vi "Expected Vertex Order.vi"(11 "Draw Mode":T1(ring)) -> (3 "Picture":picture)   [LabVIEW 2016]
doc: "Create a picture to illustrate how the mesh would use vertices to generate the 3D picture."
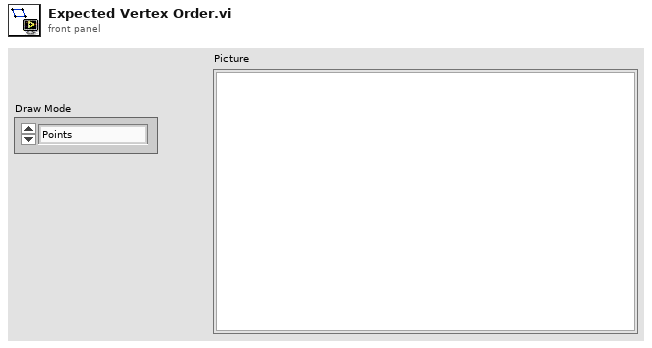
[diagram p1: front panel]
types:
  T1 = enum16{"Points", "Lines", "Line Strip", "Line Loop", "Triangles", "Triangle Strip", "Triangle Fan", "Quads", "Quad Strip", "Polygon"}
  T2 = enum16{"User-specified Font", "Application Font", "System Font", "Dialog Font"}
  T3 = cluster{"Font Name:":string, "Size":i16, "Strikeout?":bool, "Italic?":bool, "Underline?":bool, "Outline?":bool, "Shadow?":bool, "Bold?":bool}
  T4 = cluster{"Width":u16, "Style":enum32{"Solid", "Dash", "Dot", "DashDot", "DashDotDot"}}
  T5 = cluster{"horizontal":enum16{"left", "center", "right"}, "vertical":enum16{"top", "center", "bottom"}}
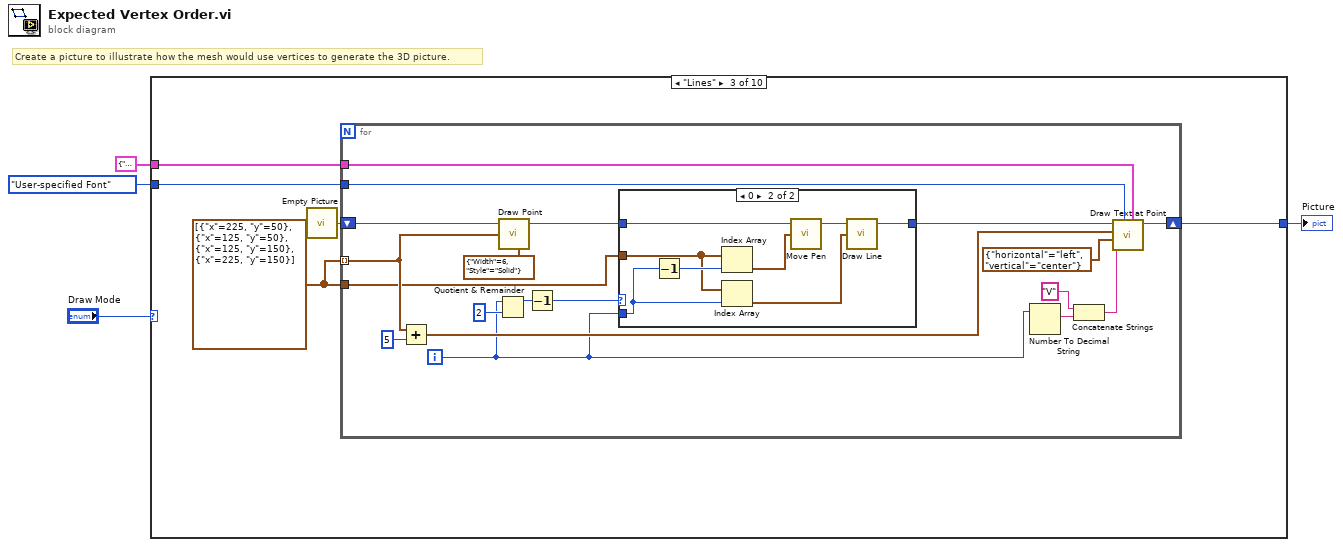
[diagram p0: block diagram]
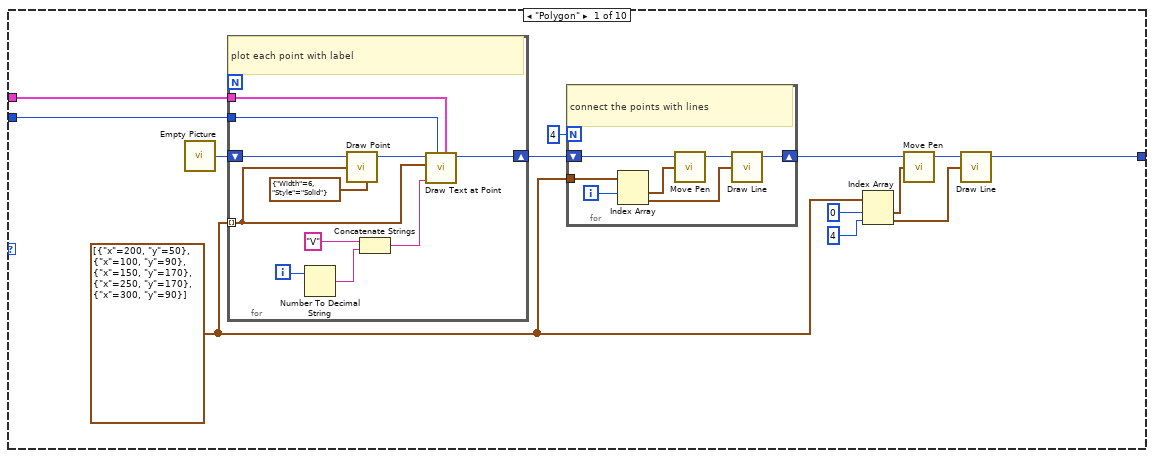
[diagram p2: hidden frame]
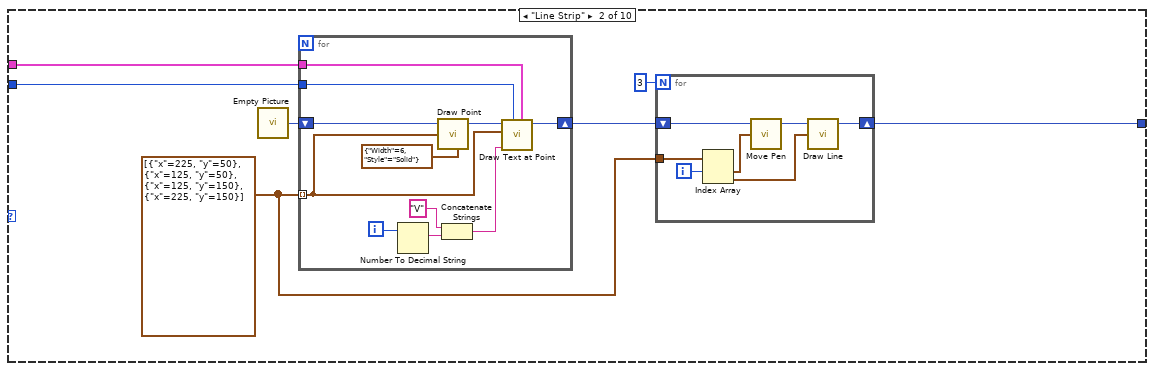
[diagram p3: hidden frame]
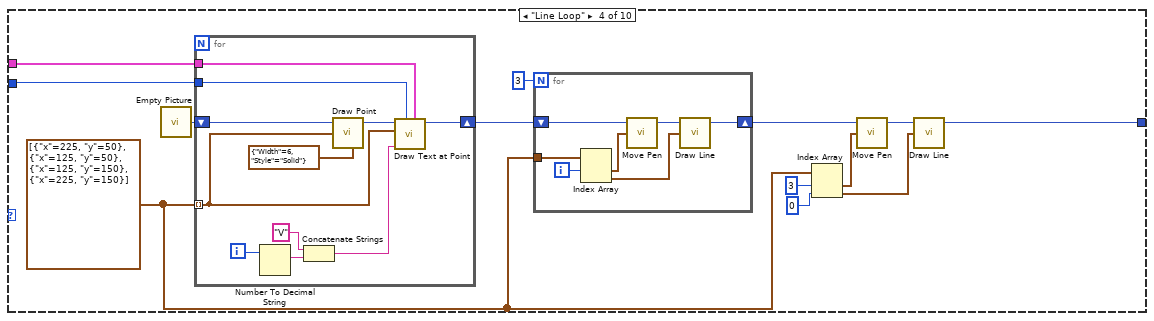
[diagram p5: hidden frame]
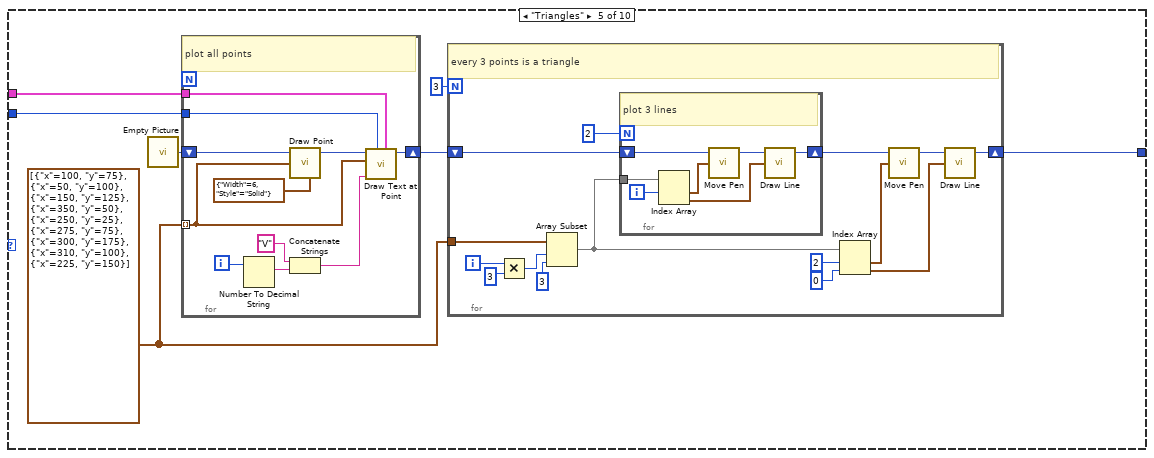
[diagram p6: hidden frame]
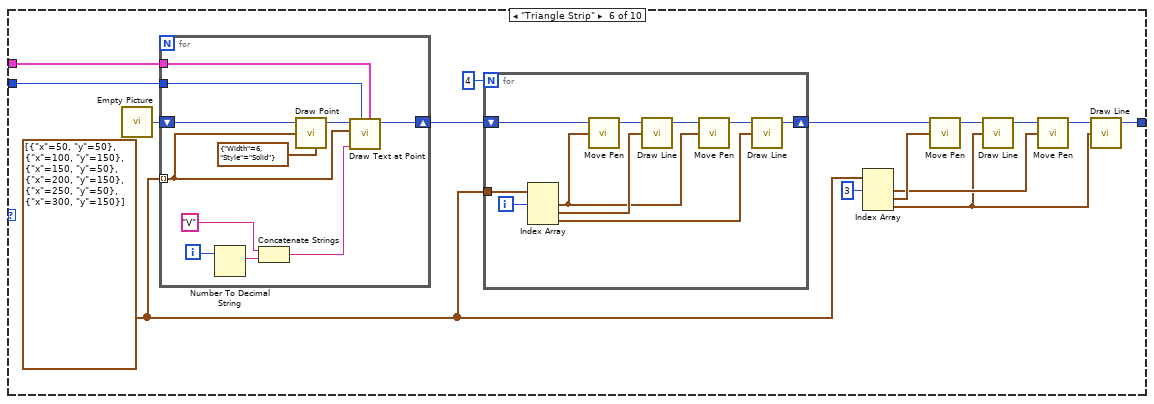
[diagram p7: hidden frame]
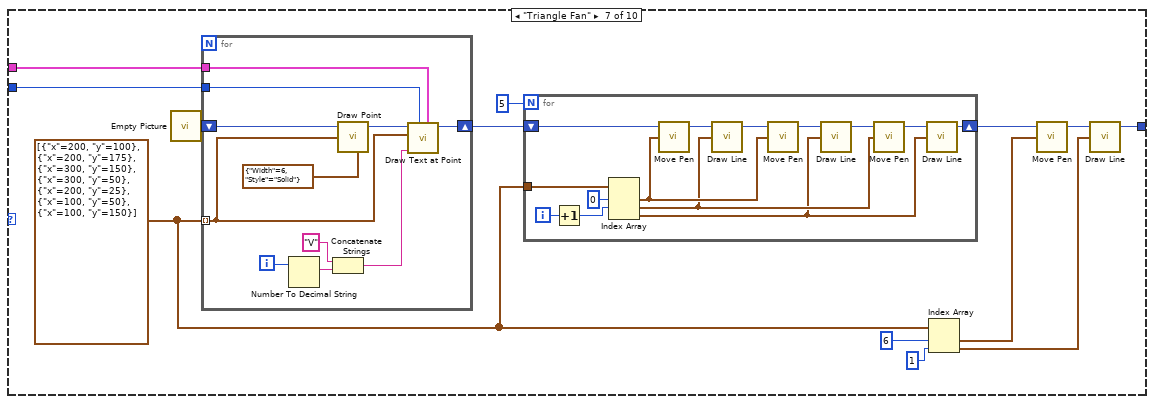
[diagram p8: hidden frame]
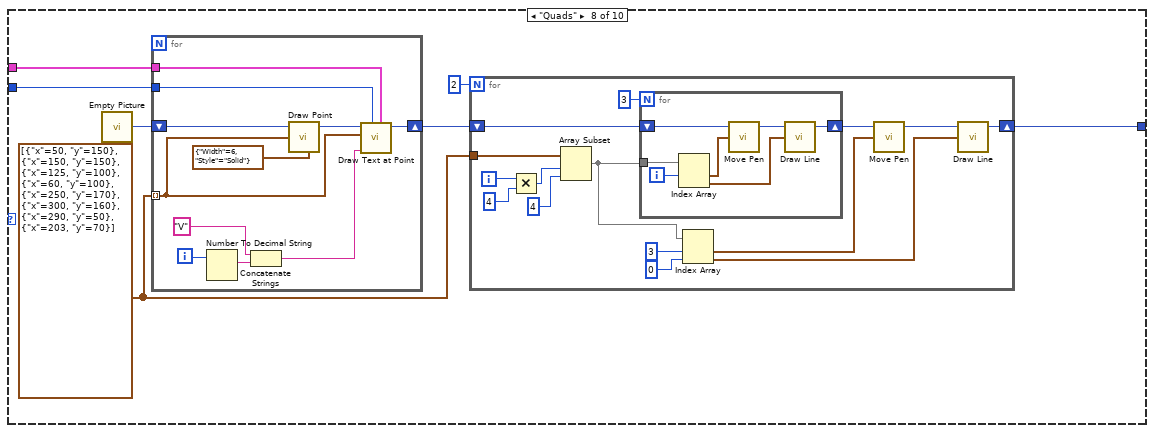
[diagram p9: hidden frame]
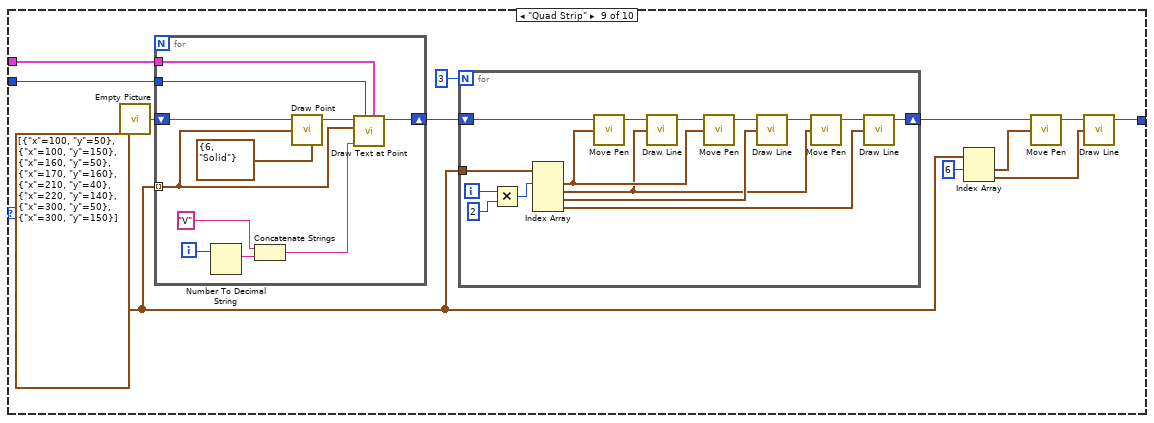
[diagram p10: hidden frame]
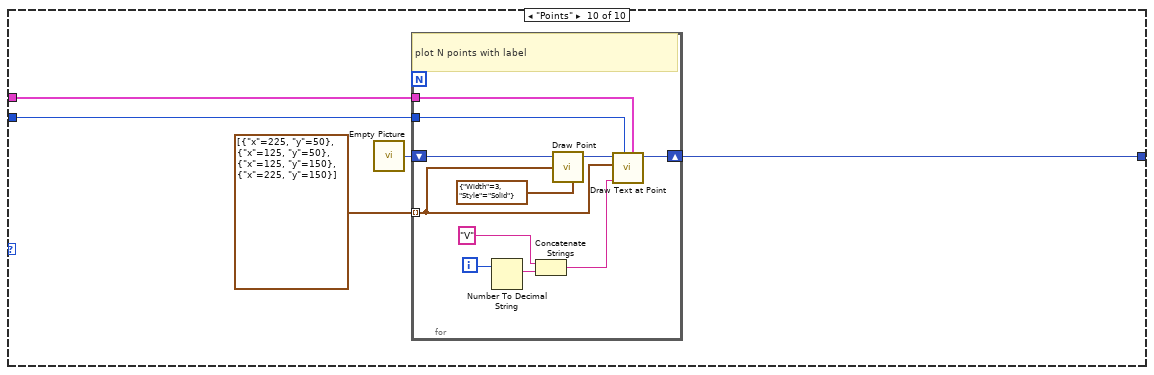
[diagram p11: hidden frame]
diagram:
  # "Create a picture to illustrate how the mesh would use vertices to generate the 3D picture."
  n1 = case shown="\"Lines\"" "Draw Mode" {
    tunnel: [w7 w38 w64 w101 w127 w170 w208 w241 w282 w320] -> w3
    tunnel: T3 {"Font Name:"="Courier", "Size"=15, "Strikeout?"=FALSE, "Italic?"=FALSE, "Underline?"=FALSE, "Outline?"=FALSE, "Shadow?"=FALSE, "Bold?"=TRUE} ("[user-specified font]") -> [w6 w36 w62 w94 w126 w165 w202 w240 w281 w317]
    tunnel: T2."User-specified Font" ("desired font(Application)") -> [w5 w37 w61 w95 w125 w166 w203 w239 w280 w318]
    frame "Polygon" {
      w10 = cluster{"x":i16, "y":i16}[] [{"x"=200, "y"=50}, {"x"=100, "y"=90}, {"x"=150, "y"=170}, {"x"=250, "y"=170}, {"x"=300, "y"=90}]
      n2 = call "Empty Picture"() -> ("empty picture"=w17:picture)
      n3 = for {
        tunnel: w10 -> [w35] mode=indexing
        shift-right: [w27] -> w15
        shift-left: w17 -> [w29]
        tunnel: w6 -> [w26]
        tunnel: w5 -> [w25]
        i -> [w33]
        # "plot each point with label"
        n4 = Number To Decimal String(number=w33) -> (decimal integer string=w32:string)  [unwired: 1 in]
        n5 = call <vilib>:"Draw Point.vi"("picture"=w29, "point(x,y)"=w35, "pen"=T4 {"Width"=6, "Style"=enum."Solid"}) -> ("new picture"=w28:picture)  [unwired: 6 in]
        n6 = Concatenate Strings("V", w32) -> (w30:string)
        n7 = call <vilib>:"Draw Text at Point.vi"("[user-specified font]"=w26, "desired font(Application)"=w25, "text"=w30, "origin"=w35, "picture"=w28) -> ("new picture"=w27:picture)  [unwired: 5 in, 1 out]
      }
      n8 = for {
        N: 4 -> [_]
        shift-right: [w20] -> w11
        shift-left: w15 -> [w21]
        tunnel: w10 -> [w19]
        i -> [w18]
        # "connect the points with lines"
        n9 = Index Array(array=w19, index #1=w18) -> (element #1=w24:cluster{"x":i16, "y":i16}, element #2=w23:cluster{"x":i16, "y":i16})  [unwired: 1 in]
        n10 = call <vilib>:"Move Pen.vi"("new position"=w24, "picture"=w21) -> ("new picture"=w22:picture)  [unwired: 3 in]
        n11 = call <vilib>:"Draw Line.vi"("picture"=w22, "end point"=w23) -> ("new picture"=w20:picture)  [unwired: 7 in]
      }
      n12 = Index Array(array=w10, index #1=0 ("index"), index #2=4 ("index")) -> (element #1=w12:cluster{"x":i16, "y":i16}, element #2=w13:cluster{"x":i16, "y":i16})
      n13 = call <vilib>:"Move Pen.vi"("new position"=w12, "picture"=w11) -> ("new picture"=w14:picture)  [unwired: 3 in]
      n14 = call <vilib>:"Draw Line.vi"("picture"=w14, "end point"=w13) -> ("new picture"=w7:picture)  [unwired: 7 in]
    }
    frame "Line Strip" {
      w39 = cluster{"x":i16, "y":i16}[] [{"x"=225, "y"=50}, {"x"=125, "y"=50}, {"x"=125, "y"=150}, {"x"=225, "y"=150}]
      n15 = call "Empty Picture"() -> ("empty picture"=w42:picture)
      n16 = for {
        tunnel: w39 -> [w60] mode=indexing
        shift-right: [w52] -> w41
        shift-left: w42 -> [w54]
        tunnel: w37 -> [w51]
        tunnel: w36 -> [w50]
        i -> [w58]
        n17 = Number To Decimal String(number=w58) -> (decimal integer string=w57:string)  [unwired: 1 in]
        n18 = call <vilib>:"Draw Point.vi"("picture"=w54, "point(x,y)"=w60, "pen"=T4 {"Width"=6, "Style"=enum."Solid"}) -> ("new picture"=w53:picture)  [unwired: 6 in]
        n19 = Concatenate Strings("V", w57) -> (w55:string)
        n20 = call <vilib>:"Draw Text at Point.vi"("[user-specified font]"=w50, "desired font(Application)"=w51, "text"=w55, "origin"=w60, "picture"=w53) -> ("new picture"=w52:picture)  [unwired: 5 in, 1 out]
      }
      n21 = for {
        N: 3 -> [_]
        shift-right: [w43] -> w38
        shift-left: w41 -> [w44]
        tunnel: w39 -> [w48]
        i -> [w49]
        n22 = Index Array(array=w48, index #1=w49) -> (element #1=w47:cluster{"x":i16, "y":i16}, element #2=w46:cluster{"x":i16, "y":i16})  [unwired: 1 in]
        n23 = call <vilib>:"Move Pen.vi"("new position"=w47, "picture"=w44) -> ("new picture"=w45:picture)  [unwired: 3 in]
        n24 = call <vilib>:"Draw Line.vi"("picture"=w45, "end point"=w46) -> ("new picture"=w43:picture)  [unwired: 7 in]
      }
    }
    frame "Lines" {
      w63 = cluster{"x":i16, "y":i16}[] [{"x"=225, "y"=50}, {"x"=125, "y"=50}, {"x"=125, "y"=150}, {"x"=225, "y"=150}]
      n25 = call "Empty Picture"() -> ("empty picture"=w65:picture)
      n26 = for {
        tunnel: w63 -> [w84] mode=indexing
        shift-right: [w78] -> w64
        shift-left: w65 -> [w79]
        tunnel: w63 -> [w72]
        tunnel: w62 -> [w68]
        tunnel: w61 -> [w67]
        i -> [w71]
        n27 = Add(x=w84, y=5) -> (x+y=w75:cluster{"x":i32, "y":i32})
        n28 = Quotient & Remainder(x=w71, y=2) -> (x-y*floor(x/y)=w73:i32)  [unwired: 1 out]
        n29 = call <vilib>:"Draw Point.vi"("picture"=w79, "point(x,y)"=w84, "pen"=T4 {"Width"=6, "Style"=enum."Solid"}) -> ("new picture"=w70:picture)  [unwired: 6 in]
        n30 = Decrement(x=w73) -> (x-1=w66:i32)
        n31 = case shown="0" w66 {
          tunnel: w72 -> [_ w90]
          tunnel: w71 -> [_ w89]
          tunnel: w70 -> [w85 w91]
          tunnel: [w85 w86] -> w69
          frame Default {
          }
          frame 0 {
            n32 = Decrement(x=w89) -> (x-1=w93:i32)
            n33 = Index Array(array=w90, index=w93) -> (element=w92:cluster{"x":i16, "y":i16})
            n34 = Index Array(array=w90, index=w89) -> (element=w88:cluster{"x":i16, "y":i16})
            n35 = call <vilib>:"Move Pen.vi"("new position"=w92, "picture"=w91) -> ("new picture"=w87:picture)  [unwired: 3 in]
            n36 = call <vilib>:"Draw Line.vi"("picture"=w87, "end point"=w88) -> ("new picture"=w86:picture)  [unwired: 7 in]
          }
        }
        n37 = Number To Decimal String(number=w71) -> (decimal integer string=w82:string)  [unwired: 1 in]
        n38 = Concatenate Strings("V", w82) -> (w80:string)
        n39 = call <vilib>:"Draw Text at Point.vi"("[user-specified font]"=w68, "desired font(Application)"=w67, "text"=w80, "alignment(left, top)"=T5 {"horizontal"=enum."left", "vertical"=enum."center"}, "origin"=w75, "picture"=w69) -> ("new picture"=w78:picture)  [unwired: 4 in, 1 out]
      }
    }
    frame "Line Loop" {
      w98 = cluster{"x":i16, "y":i16}[] [{"x"=225, "y"=50}, {"x"=125, "y"=50}, {"x"=125, "y"=150}, {"x"=225, "y"=150}]
      n40 = call "Empty Picture"() -> ("empty picture"=w106:picture)
      n41 = for {
        tunnel: w98 -> [w124] mode=indexing
        shift-right: [w116] -> w104
        shift-left: w106 -> [w118]
        tunnel: w95 -> [w115]
        tunnel: w94 -> [w114]
        i -> [w122]
        n42 = Number To Decimal String(number=w122) -> (decimal integer string=w121:string)  [unwired: 1 in]
        n43 = Concatenate Strings("V", w121) -> (w119:string)
        n44 = call <vilib>:"Draw Point.vi"("picture"=w118, "point(x,y)"=w124, "pen"=T4 {"Width"=6, "Style"=enum."Solid"}) -> ("new picture"=w117:picture)  [unwired: 6 in]
        n45 = call <vilib>:"Draw Text at Point.vi"("[user-specified font]"=w114, "desired font(Application)"=w115, "text"=w119, "origin"=w124, "picture"=w117) -> ("new picture"=w116:picture)  [unwired: 5 in, 1 out]
      }
      n46 = for {
        N: 3 -> [_]
        shift-right: [w107] -> w102
        shift-left: w104 -> [w108]
        tunnel: w98 -> [w112]
        i -> [w113]
        n47 = Index Array(array=w112, index #1=w113) -> (element #1=w111:cluster{"x":i16, "y":i16}, element #2=w110:cluster{"x":i16, "y":i16})  [unwired: 1 in]
        n48 = call <vilib>:"Move Pen.vi"("new position"=w111, "picture"=w108) -> ("new picture"=w109:picture)  [unwired: 3 in]
        n49 = call <vilib>:"Draw Line.vi"("picture"=w109, "end point"=w110) -> ("new picture"=w107:picture)  [unwired: 7 in]
      }
      n50 = Index Array(array=w98, index #1=3 ("index"), index #2=0 ("index")) -> (element #1=w97:cluster{"x":i16, "y":i16}, element #2=w96:cluster{"x":i16, "y":i16})
      n51 = call <vilib>:"Move Pen.vi"("new position"=w97, "picture"=w102) -> ("new picture"=w103:picture)  [unwired: 3 in]
      n52 = call <vilib>:"Draw Line.vi"("picture"=w103, "end point"=w96) -> ("new picture"=w101:picture)  [unwired: 7 in]
    }
    frame "Triangles" {
      w129 = cluster{"x":i16, "y":i16}[] [{"x"=100, "y"=75}, {"x"=50, "y"=100}, {"x"=150, "y"=125}, {"x"=350, "y"=50}, {"x"=250, "y"=25}, {"x"=275, "y"=75}, {"x"=300, "y"=175}, {"x"=310, "y"=100}, {"x"=225, "y"=150}]
      n53 = call "Empty Picture"() -> ("empty picture"=w131:picture)
      n54 = for {
        tunnel: w129 -> [w164] mode=indexing
        shift-right: [w156] -> w128
        shift-left: w131 -> [w158]
        tunnel: w126 -> [w155]
        tunnel: w125 -> [w154]
        i -> [w162]
        # "plot all points"
        n55 = Number To Decimal String(number=w162) -> (decimal integer string=w161:string)  [unwired: 1 in]
        n56 = call <vilib>:"Draw Point.vi"("picture"=w158, "point(x,y)"=w164, "pen"=T4 {"Width"=6, "Style"=enum."Solid"}) -> ("new picture"=w157:picture)  [unwired: 6 in]
        n57 = Concatenate Strings("V", w161) -> (w159:string)
        n58 = call <vilib>:"Draw Text at Point.vi"("[user-specified font]"=w155, "desired font(Application)"=w154, "text"=w159, "origin"=w164, "picture"=w157) -> ("new picture"=w156:picture)  [unwired: 5 in, 1 out]
      }
      n59 = for {
        N: 3 -> [_]
        tunnel: w129 -> [w143]
        shift-right: [w133] -> w127
        shift-left: w128 -> [w140]
        i -> [w146]
        # "every 3 points is a triangle"
        n60 = Multiply(x=w146, y=3) -> (x*y=w144:i32)
        n61 = Array Subset(array=w143, index=w144, length=3) -> (w139:cluster{"x":i16, "y":i16}[])
        n62 = for {
          N: 2 -> [_]
          tunnel: w139 -> [w153]
          shift-right: [w147] -> w136
          shift-left: w140 -> [w148]
          i -> [w152]
          # "plot 3 lines"
          n63 = Index Array(array=w153, index #1=w152) -> (element #1=w151:cluster{"x":i16, "y":i16}, element #2=w149:cluster{"x":i16, "y":i16})  [unwired: 1 in]
          n64 = call <vilib>:"Move Pen.vi"("new position"=w151, "picture"=w148) -> ("new picture"=w150:picture)  [unwired: 3 in]
          n65 = call <vilib>:"Draw Line.vi"("picture"=w150, "end point"=w149) -> ("new picture"=w147:picture)  [unwired: 7 in]
        }
        n66 = Index Array(array=w139, index #1=2 ("index"), index #2=0 ("index")) -> (element #1=w135:cluster{"x":i16, "y":i16}, element #2=w134:cluster{"x":i16, "y":i16})
        n67 = call <vilib>:"Move Pen.vi"("new position"=w135, "picture"=w136) -> ("new picture"=w137:picture)  [unwired: 3 in]
        n68 = call <vilib>:"Draw Line.vi"("picture"=w137, "end point"=w134) -> ("new picture"=w133:picture)  [unwired: 7 in]
      }
    }
    frame "Triangle Strip" {
      w174 = cluster{"x":i16, "y":i16}[] [{"x"=50, "y"=50}, {"x"=100, "y"=150}, {"x"=150, "y"=50}, {"x"=200, "y"=150}, {"x"=250, "y"=50}, {"x"=300, "y"=150}]
      n69 = call "Empty Picture"() -> ("empty picture"=w179:picture)
      n70 = for {
        tunnel: w174 -> [w200] mode=indexing
        shift-right: [w192] -> w177
        shift-left: w179 -> [w194]
        tunnel: w166 -> [w191]
        tunnel: w165 -> [w190]
        i -> [w198]
        n71 = Number To Decimal String(number=w198) -> (decimal integer string=w197:string)  [unwired: 1 in]
        n72 = Concatenate Strings("V", w197) -> (w195:string)
        n73 = call <vilib>:"Draw Point.vi"("picture"=w194, "point(x,y)"=w200, "pen"=T4 {"Width"=6, "Style"=enum."Solid"}) -> ("new picture"=w193:picture)  [unwired: 6 in]
        n74 = call <vilib>:"Draw Text at Point.vi"("[user-specified font]"=w190, "desired font(Application)"=w191, "text"=w195, "origin"=w200, "picture"=w193) -> ("new picture"=w192:picture)  [unwired: 5 in, 1 out]
      }
      n75 = for {
        N: 4 -> [_]
        shift-right: [w181] -> w175
        shift-left: w177 -> [w187]
        tunnel: w174 -> [w189]
        i -> [w188]
        n76 = Index Array(array=w189, index #1=w188) -> (element #1=w183:cluster{"x":i16, "y":i16}, element #2=w185:cluster{"x":i16, "y":i16}, element #3=w180:cluster{"x":i16, "y":i16})  [unwired: 2 in]
        n77 = call <vilib>:"Move Pen.vi"("new position"=w183, "picture"=w187) -> ("new picture"=w186:picture)  [unwired: 3 in]
        n78 = call <vilib>:"Draw Line.vi"("picture"=w186, "end point"=w185) -> ("new picture"=w184:picture)  [unwired: 7 in]
        n79 = call <vilib>:"Move Pen.vi"("new position"=w183, "picture"=w184) -> ("new picture"=w182:picture)  [unwired: 3 in]
        n80 = call <vilib>:"Draw Line.vi"("picture"=w182, "end point"=w180) -> ("new picture"=w181:picture)  [unwired: 7 in]
      }
      n81 = Index Array(array=w174, index #1=3 ("index")) -> (element #1=w168:cluster{"x":i16, "y":i16}, element #2=w172:cluster{"x":i16, "y":i16}, element #3=w167:cluster{"x":i16, "y":i16})  [unwired: 2 in]
      n82 = call <vilib>:"Move Pen.vi"("new position"=w172, "picture"=w175) -> ("new picture"=w176:picture)  [unwired: 3 in]
      n83 = call <vilib>:"Draw Line.vi"("picture"=w176, "end point"=w167) -> ("new picture"=w169:picture)  [unwired: 7 in]
      n84 = call <vilib>:"Move Pen.vi"("new position"=w168, "picture"=w169) -> ("new picture"=w171:picture)  [unwired: 3 in]
      n85 = call <vilib>:"Draw Line.vi"("picture"=w171, "end point"=w167) -> ("new picture"=w170:picture)  [unwired: 7 in]
    }
    frame "Triangle Fan" {
      w201 = cluster{"x":i16, "y":i16}[] [{"x"=200, "y"=100}, {"x"=200, "y"=175}, {"x"=300, "y"=150}, {"x"=300, "y"=50}, {"x"=200, "y"=25}, {"x"=100, "y"=50}, {"x"=100, "y"=150}]
      n86 = call "Empty Picture"() -> ("empty picture"=w213:picture)
      n87 = for {
        tunnel: w201 -> [w238] mode=indexing
        shift-right: [w230] -> w212
        shift-left: w213 -> [w232]
        tunnel: w203 -> [w229]
        tunnel: w202 -> [w228]
        i -> [w236]
        n88 = Number To Decimal String(number=w236) -> (decimal integer string=w235:string)  [unwired: 1 in]
        n89 = Concatenate Strings("V", w235) -> (w233:string)
        n90 = call <vilib>:"Draw Point.vi"("picture"=w232, "point(x,y)"=w238, "pen"=T4 {"Width"=6, "Style"=enum."Solid"}) -> ("new picture"=w231:picture)  [unwired: 6 in]
        n91 = call <vilib>:"Draw Text at Point.vi"("[user-specified font]"=w228, "desired font(Application)"=w229, "text"=w233, "origin"=w238, "picture"=w231) -> ("new picture"=w230:picture)  [unwired: 5 in, 1 out]
      }
      n92 = for {
        N: 5 -> [_]
        shift-right: [w218] -> w209
        shift-left: w212 -> [w219]
        tunnel: w201 -> [w227]
        i -> [w216]
        n93 = Increment(x=w216) -> (x+1=w215:i32)
        n94 = Index Array(array=w227, index #1=0 ("index"), index #2=w215) -> (element #1=w223:cluster{"x":i16, "y":i16}, element #2=w222:cluster{"x":i16, "y":i16}, element #3=w217:cluster{"x":i16, "y":i16})  [unwired: 1 in]
        n95 = call <vilib>:"Move Pen.vi"("new position"=w223, "picture"=w219) -> ("new picture"=w226:picture)  [unwired: 3 in]
        n96 = call <vilib>:"Draw Line.vi"("picture"=w226, "end point"=w222) -> ("new picture"=w220:picture)  [unwired: 7 in]
        n97 = call <vilib>:"Move Pen.vi"("new position"=w223, "picture"=w220) -> ("new picture"=w225:picture)  [unwired: 3 in]
        n98 = call <vilib>:"Draw Line.vi"("picture"=w225, "end point"=w217) -> ("new picture"=w221:picture)  [unwired: 7 in]
        n99 = call <vilib>:"Move Pen.vi"("new position"=w222, "picture"=w221) -> ("new picture"=w224:picture)  [unwired: 3 in]
        n100 = call <vilib>:"Draw Line.vi"("picture"=w224, "end point"=w217) -> ("new picture"=w218:picture)  [unwired: 7 in]
      }
      n101 = Index Array(array=w201, index #1=6 ("index"), index #2=1 ("index")) -> (element #1=w205:cluster{"x":i16, "y":i16}, element #2=w204:cluster{"x":i16, "y":i16})
      n102 = call <vilib>:"Move Pen.vi"("new position"=w205, "picture"=w209) -> ("new picture"=w210:picture)  [unwired: 3 in]
      n103 = call <vilib>:"Draw Line.vi"("picture"=w210, "end point"=w204) -> ("new picture"=w208:picture)  [unwired: 7 in]
    }
    frame "Quads" {
      w242 = cluster{"x":i16, "y":i16}[] [{"x"=50, "y"=150}, {"x"=150, "y"=150}, {"x"=125, "y"=100}, {"x"=60, "y"=100}, {"x"=250, "y"=170}, {"x"=300, "y"=160}, {"x"=290, "y"=50}, {"x"=203, "y"=70}]
      n104 = call "Empty Picture"() -> ("empty picture"=w245:picture)
      n105 = for {
        tunnel: w242 -> [w278] mode=indexing
        shift-right: [w270] -> w243
        shift-left: w245 -> [w272]
        tunnel: w240 -> [w269]
        tunnel: w239 -> [w268]
        i -> [w276]
        n106 = Number To Decimal String(number=w276) -> (decimal integer string=w275:string)  [unwired: 1 in]
        n107 = Concatenate Strings("V", w275) -> (w273:string)
        n108 = call <vilib>:"Draw Point.vi"("picture"=w272, "point(x,y)"=w278, "pen"=T4 {"Width"=6, "Style"=enum."Solid"}) -> ("new picture"=w271:picture)  [unwired: 6 in]
        n109 = call <vilib>:"Draw Text at Point.vi"("[user-specified font]"=w269, "desired font(Application)"=w268, "text"=w273, "origin"=w278, "picture"=w271) -> ("new picture"=w270:picture)  [unwired: 5 in, 1 out]
      }
      n110 = for {
        N: 2 -> [_]
        shift-right: [w248] -> w241
        shift-left: w243 -> [w249]
        tunnel: w242 -> [w258]
        i -> [w260]
        n111 = Multiply(x=w260, y=4) -> (x*y=w257:i32)
        n112 = Array Subset(array=w258, index=w257, length=4) -> (w247:cluster{"x":i16, "y":i16}[])
        n113 = for {
          N: 3 -> [_]
          tunnel: w247 -> [w267]
          shift-right: [w261] -> w252
          shift-left: w249 -> [w262]
          i -> [w266]
          n114 = Index Array(array=w267, index #1=w266) -> (element #1=w265:cluster{"x":i16, "y":i16}, element #2=w263:cluster{"x":i16, "y":i16})  [unwired: 1 in]
          n115 = call <vilib>:"Move Pen.vi"("new position"=w265, "picture"=w262) -> ("new picture"=w264:picture)  [unwired: 3 in]
          n116 = call <vilib>:"Draw Line.vi"("picture"=w264, "end point"=w263) -> ("new picture"=w261:picture)  [unwired: 7 in]
        }
        n117 = Index Array(array=w247, index #1=3 ("index"), index #2=0 ("index")) -> (element #1=w251:cluster{"x":i16, "y":i16}, element #2=w250:cluster{"x":i16, "y":i16})
        n118 = call <vilib>:"Move Pen.vi"("new position"=w251, "picture"=w252) -> ("new picture"=w253:picture)  [unwired: 3 in]
        n119 = call <vilib>:"Draw Line.vi"("picture"=w253, "end point"=w250) -> ("new picture"=w248:picture)  [unwired: 7 in]
      }
    }
    frame "Quad Strip" {
      w279 = cluster{"x":i16, "y":i16}[] [{"x"=100, "y"=50}, {"x"=100, "y"=150}, {"x"=160, "y"=50}, {"x"=170, "y"=160}, {"x"=210, "y"=40}, {"x"=220, "y"=140}, {"x"=300, "y"=50}, {"x"=300, "y"=150}]
      n120 = call "Empty Picture"() -> ("empty picture"=w290:picture)
      n121 = for {
        tunnel: w279 -> [w316] mode=indexing
        shift-right: [w308] -> w285
        shift-left: w290 -> [w310]
        tunnel: w281 -> [w307]
        tunnel: w280 -> [w306]
        i -> [w314]
        n122 = Number To Decimal String(number=w314) -> (decimal integer string=w313:string)  [unwired: 1 in]
        n123 = Concatenate Strings("V", w313) -> (w311:string)
        n124 = call <vilib>:"Draw Point.vi"("picture"=w310, "point(x,y)"=w316, "pen"=T4 {"Width"=6, "Style"=enum."Solid"}) -> ("new picture"=w309:picture)  [unwired: 6 in]
        n125 = call <vilib>:"Draw Text at Point.vi"("[user-specified font]"=w307, "desired font(Application)"=w306, "text"=w311, "origin"=w316, "picture"=w309) -> ("new picture"=w308:picture)  [unwired: 5 in, 1 out]
      }
      n126 = for {
        N: 3 -> [_]
        shift-right: [w296] -> w287
        shift-left: w285 -> [w303]
        tunnel: w279 -> [w305]
        i -> [w304]
        n127 = Multiply(x=w304, y=2) -> (x*y=w294:i32)
        n128 = Index Array(array=w305, index #1=w294) -> (element #1=w300:cluster{"x":i16, "y":i16}, element #2=w292:cluster{"x":i16, "y":i16}, element #3=w298:cluster{"x":i16, "y":i16}, element #4=w291:cluster{"x":i16, "y":i16})  [unwired: 3 in]
        n129 = call <vilib>:"Move Pen.vi"("new position"=w300, "picture"=w303) -> ("new picture"=w302:picture)  [unwired: 3 in]
        n130 = call <vilib>:"Draw Line.vi"("picture"=w302, "end point"=w292) -> ("new picture"=w301:picture)  [unwired: 7 in]
        n131 = call <vilib>:"Move Pen.vi"("new position"=w300, "picture"=w301) -> ("new picture"=w299:picture)  [unwired: 3 in]
        n132 = call <vilib>:"Draw Line.vi"("picture"=w299, "end point"=w298) -> ("new picture"=w295:picture)  [unwired: 7 in]
        n133 = call <vilib>:"Move Pen.vi"("new position"=w292, "picture"=w295) -> ("new picture"=w297:picture)  [unwired: 3 in]
        n134 = call <vilib>:"Draw Line.vi"("picture"=w297, "end point"=w291) -> ("new picture"=w296:picture)  [unwired: 7 in]
      }
      n135 = Index Array(array=w279, index #1=6 ("index")) -> (element #1=w284:cluster{"x":i16, "y":i16}, element #2=w283:cluster{"x":i16, "y":i16})  [unwired: 1 in]
      n136 = call <vilib>:"Move Pen.vi"("new position"=w284, "picture"=w287) -> ("new picture"=w288:picture)  [unwired: 3 in]
      n137 = call <vilib>:"Draw Line.vi"("picture"=w288, "end point"=w283) -> ("new picture"=w282:picture)  [unwired: 7 in]
    }
    frame "Points" {
      n138 = call "Empty Picture"() -> ("empty picture"=w321:picture)
      n139 = for {
        tunnel: cluster{"x":i16, "y":i16}[] [{"x"=225, "y"=50}, {"x"=125, "y"=50}, {"x"=125, "y"=150}, {"x"=225, "y"=150}] -> [w332] mode=indexing
        shift-right: [w324] -> w320
        shift-left: w321 -> [w326]
        tunnel: w318 -> [w323]
        tunnel: w317 -> [w322]
        i -> [w330]
        # "plot N points with label"
        n140 = Number To Decimal String(number=w330) -> (decimal integer string=w329:string)  [unwired: 1 in]
        n141 = Concatenate Strings("V", w329) -> (w327:string)
        n142 = call <vilib>:"Draw Point.vi"("picture"=w326, "point(x,y)"=w332, "pen"=T4 {"Width"=3, "Style"=enum."Solid"}) -> ("new picture"=w325:picture)  [unwired: 6 in]
        n143 = call <vilib>:"Draw Text at Point.vi"("[user-specified font]"=w322, "desired font(Application)"=w323, "text"=w327, "origin"=w332, "picture"=w325) -> ("new picture"=w324:picture)  [unwired: 5 in, 1 out]
      }
    }
  }
  "Picture" <- w3
